vi "DAQmx Create Channel (TEDS-AI-Temperature-RTD).vi"(0 "task in":refnum<k21>, 1 "maximum value":dbl=100.0 format="%0.2f", 2 "minimum value":dbl format="%0.2f", 3 "resistance configuration":i32(ring)=2 items=["2-Wire"=2, "3-Wire"=3, "4-Wire"=4], 5 "physical channels":tag, 7 "name to assign":string, 9 "units":i32(ring)=10143 items=["Deg C"=10143, "Deg F"=10144, "Kelvins"=10325, "Deg R"=10145, "From Custom Scale"=10065], 10 "current excitation value":dbl=0.0025 format="%0.5f", 11 "error in":errorcluster, 13 "current excitation source":i32(ring)=10167 items=["Internal"=10200, "External"=10167, "None"=10230]) -> (4 "task out":refnum<k21>, 15 "error out":errorcluster)   [LabVIEW 2011]
doc: "Creates channel(s) that use an RTD to measure temperature. You must configure the physical channel(s) with TEDS information to use this VI."
uses:
  C:/Program Files/National Instruments/LabVIEW 2011/resource/objmgr/daqmx.rc
panel:
  # "input limits"
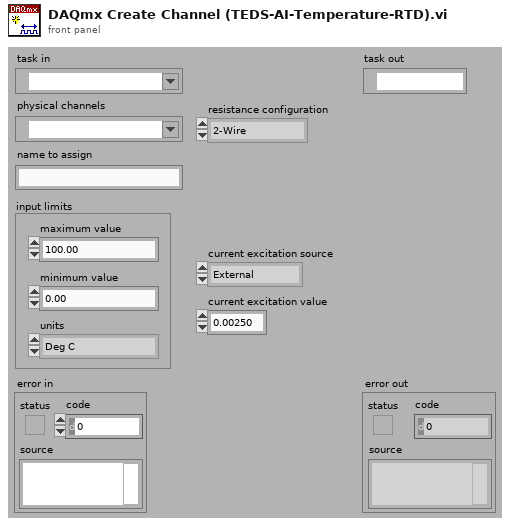
[diagram p1: front panel]
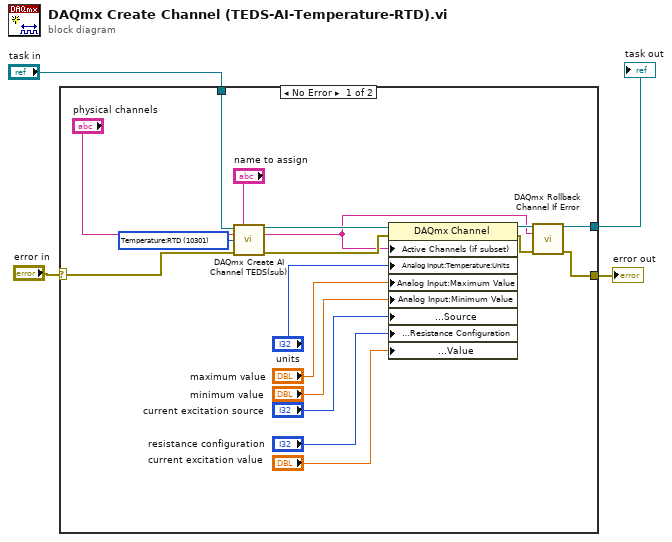
[diagram p0: block diagram]
diagram:
  n1 = case shown="No Error" "error in" {
    selector: "error in" -> [w21 w23]
    tunnel: [w8 w23] -> w4
    tunnel: "task in" -> [w22 w24]
    tunnel: [w7 w24] -> w1
    frame No Error {
      w5 = 10301 items=["Voltage"=10322, "Current"=10134, "More:Voltage:Custom with Excitation"=10323, "More:Current:Custom with Excitation"=10136, "Frequency"=10181, "Period"=10257, "Resistance"=10278, "Temperature:Thermocouple"=10303, "Temperature:Thermistor"=10302, "Temperature:RTD"=10301, "Temperature:Built-in Sensor"=10311, "Strain Gage"=10300, "LVDT"=10352, "RVDT"=10353, "Accelerometer:Voltage Input"=10355, "Accelerometer:Current Input"=10356, "Sound Pressure:Microphone"=10354, "TEDS"=12531] ("measurement type")
      n2 = call "DAQmx Create AI Channel TEDS(sub).vi"("task in"=w22, "virtual channel name"="name to assign", "physical channel name"="physical channels", "measurement type"=w5, "error in"=w21) -> ("task out"=w11:refnum<k21>, "channel names"=w6:string, "error out"=w19:errorcluster)  [unwired: 1 in, 7 out]
      n3 = property class="DAQmx Channel"(reference=w11, error in=w19, "Active Channels (if subset)"=w6, "Analog Input:Temperature:Units"="units", "Analog Input:Maximum Value"="maximum value", "Analog Input:Minimum Value"="minimum value", "Analog Input:General Properties:Signal Conditioning:Excitation:Source"="current excitation source", "Analog Input:General Properties:Signal Conditioning:Resistance Configuration"="resistance configuration", "Analog Input:General Properties:Signal Conditioning:Excitation:Value"="current excitation value") -> (reference out=w10:refnum<k21>, error out=w9:errorcluster)
      n4 = call "DAQmx Rollback Channel If Error.vi"("task in"=w10, "channel names"=w6, "error in"=w9) -> ("task out"=w7:refnum<k21>, "error out"=w8:errorcluster)  [unwired: 11 out]
    }
    frame Error {
    }
  }
  "error out" <- w4
  "task out" <- w1
